vi "Find Array High-Low Levels.vi"(8 "Error In":errorcluster, 9 "Method (Mode)":T1, 10 "# Bins (auto)":i32, 11 "Array":dbl[](array[numeric])) -> (0 "Error Out":errorcluster, 1 "Low Level":dbl format="%0.2f", 3 "High Level":dbl format="%0.2f")   [LabVIEW 2021, in "Arrays.lvlib"]
doc: "Split the array into its lower and higher 50 percentiles and computes the mode (or mean) of each part."
uses:
  Arrays.lvlib
  Fits/Square Pulse/Square Pulse Levels Type.ctl
  Histograms/Histogram Bin Position.ctl
  Histograms/Linear Histogram Options.ctl
  Histograms/Histogram Bin Option.ctl
  e09bfede-782a-433a-9cf0-25cc41a0cc0b.vi
  3c089a08-6f38-494f-b69c-1966d4ea5c7a.vi
  e09bfede-782a-433a-9cf0-25cc41a0cc0b.vi/e021cd17-e000-4244-b7f4-ec50548bdfcb.vi
  e09bfede-782a-433a-9cf0-25cc41a0cc0b.vi/b1828c6e-eb0a-43e9-a724-8b596c52e435.vi
  e09bfede-782a-433a-9cf0-25cc41a0cc0b.vi/7a6138ed-c001-4311-b538-9ba42ae7c7b1.vi
  e09bfede-782a-433a-9cf0-25cc41a0cc0b.vi/52c6b4fa-501b-4af0-803b-8bab516ca5d3.vi
  e09bfede-782a-433a-9cf0-25cc41a0cc0b.vi/d7237e10-35ab-4bcb-a0c6-4883c3f4c990.vi
  e09bfede-782a-433a-9cf0-25cc41a0cc0b.vi/5fb5dd96-3b97-4592-ba56-58181c8e7105.vi
  e09bfede-782a-433a-9cf0-25cc41a0cc0b.vi/8e13a849-a393-4484-9968-4af7b25c38d7.vi
  3c089a08-6f38-494f-b69c-1966d4ea5c7a.vi/e021cd17-e000-4244-b7f4-ec50548bdfcb.vi
  3c089a08-6f38-494f-b69c-1966d4ea5c7a.vi/b1828c6e-eb0a-43e9-a724-8b596c52e435.vi
  3c089a08-6f38-494f-b69c-1966d4ea5c7a.vi/7a6138ed-c001-4311-b538-9ba42ae7c7b1.vi
  3c089a08-6f38-494f-b69c-1966d4ea5c7a.vi/52c6b4fa-501b-4af0-803b-8bab516ca5d3.vi
  3c089a08-6f38-494f-b69c-1966d4ea5c7a.vi/d7237e10-35ab-4bcb-a0c6-4883c3f4c990.vi
  3c089a08-6f38-494f-b69c-1966d4ea5c7a.vi/5fb5dd96-3b97-4592-ba56-58181c8e7105.vi
  3c089a08-6f38-494f-b69c-1966d4ea5c7a.vi/8e13a849-a393-4484-9968-4af7b25c38d7.vi
  Time/High Resolution Timing.vi
  <userlib>/_OpenG.lib/array/array.llb/Filter 1D Array__ogtk.vi
  <userlib>/_OpenG.lib/array/array.llb/Filter 1D Array (DBL)__ogtk.vi
  <userlib>/_OpenG.lib/array/array.llb/Delete Elements from Array__ogtk.vi
  <userlib>/_OpenG.lib/array/array.llb/Delete Elements from 1D Array (DBL)__ogtk.vi
  <vilib>/Utility/error.llb/Error Cluster From Error Code.vi
  Histograms/Histogram Window.lvlib
  Math/Math.lvlib
  Fits/Fits.lvlib
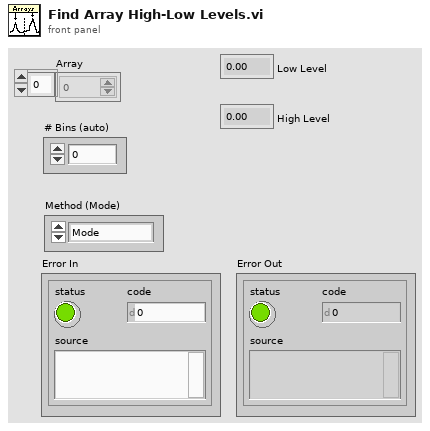
[diagram p1: front panel]
types:
  T1 = typedef "Fits.lvlib/Square Pulse Levels Type.ctl" = enum16{"Mode", "Mean"}
  T2 = typedef "Histogram Window.lvlib/Histogram Bin Option.ctl" = enum32{"Bin Number", "Bin Size"}
  T3 = typedef "Histogram Window.lvlib/Linear Histogram Options.ctl" = cluster{"Bin Size":dbl, "Bin Number":i32, "Bin Option":T2, "Min Value":dbl, "Max Value":dbl, "Filter NaN & Infinite Values":bool, "Frequency Plot":bool, "Align Bins":bool, "Bin Location":T4, "Project Outside Values":bool, "Max Histogram Size":i32}
  T4 = typedef "Histogram Window.lvlib/Histogram Bin Position.ctl" = enum16{"Left", "Center", "Right"}
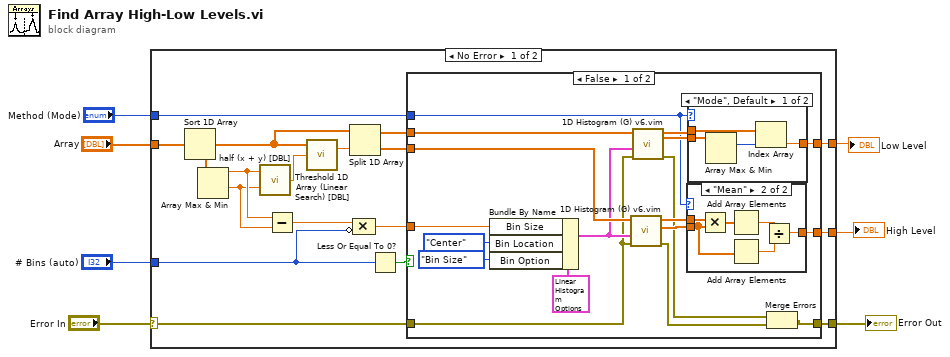
[diagram p0: block diagram]
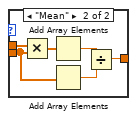
[diagram p2: hidden frame]
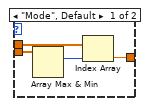
[diagram p3: hidden frame]
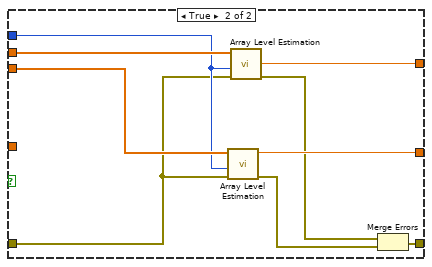
[diagram p4: hidden frame]
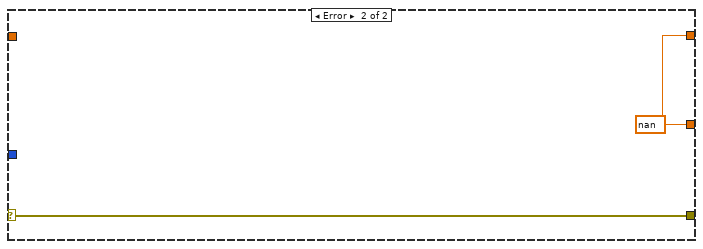
[diagram p5: hidden frame]
diagram:
  n1 = case shown="No Error" "Error In" {
    selector: "Error In" -> [w9 w73]
    tunnel: "Array" -> [w24 _]
    tunnel: [w22 w72] -> w6
    tunnel: [w21 w72] -> w5
    tunnel: "# Bins (auto)" -> [w18 _]
    tunnel: "Method (Mode)" -> [w13 _]
    tunnel: [w8 w73] -> w1
    frame No Error {
      n2 = Sort 1D Array(array=w24) -> (sorted array=w20:dbl[])
      n3 = Array Max & Min(array=w20) -> (max value=w12:dbl, min value=w11:dbl)  [unwired: 2 out]
      n4 = call "half (x + y) [DBL].vi"("y"=w11, "x"=w12) -> ("(x+y)/2"=w10:dbl)  [unwired: 4 in]
      n5 = Subtract(x=w12, y=w11) -> (x-y=w19:dbl)
      n6 = call "Threshold 1D Array (Linear Search) [DBL].vi"("Array"=w20, "Y"=w10) -> ("fractional index"=w23:dbl)  [unwired: 7 in]
      n7 = Split 1D Array(array=w20, index=w23) -> (first subarray=w14:dbl[], second subarray=w17:dbl[])
      n8 = Compound Arithmetic op=MULTIPLY(w19, invert w18) -> (w16:dbl)
      n9 = Less Or Equal To 0?(x=w18) -> (x <= 0?=w15:bool)
      n10 = case shown="False" w15 {
        tunnel: [w42 w70] -> w22
        tunnel: [w41 w71] -> w21
        tunnel: w14 -> [w36 w69]
        tunnel: w13 -> [w35 w67]
        tunnel: w17 -> [w34 w68]
        tunnel: w16 -> [w32 _]
        tunnel: w9 -> [w29 w66]
        tunnel: [w26 w63] -> w8
        frame False {
          n11 = Bundle By Name(cluster=T3 {"Bin Size"=nan, "Bin Number"=0, "Bin Option"=enum."Bin Number", "Min Value"=-inf, "Max Value"=inf, "Filter NaN & Infinite Values"=FALSE, "Frequency Plot"=FALSE, "Align Bins"=FALSE, "Bin Location"=enum."Left", "Project Outside Values"=FALSE, "Max Histogram Size"=100000} ("Histogram Options"), "Bin Size"=w32, "Bin Location"=Histogram_Bin_Position."Center" ("Bin Location (Left)"), "Bin Option"=Histogram_Bin_Option."Bin Size" ("Bin Size")) -> (w30:T3)
          n12 = call "1D Histogram (G) v6.vim"("Error In"=w29, "Histogram Options"=w30, "Array"=w34) -> ("Error Out"=w27:errorcluster, "Histogram"=w37:dbl[], "Axis"=w38:dbl[])  [unwired: 2 in, 4 out]
          n13 = call "1D Histogram (G) v6.vim"("Error In"=w29, "Histogram Options"=w30, "Array"=w36) -> ("Error Out"=w28:errorcluster, "Histogram"=w39:dbl[], "Axis"=w40:dbl[])  [unwired: 2 in, 4 out]
          n14 = case shown="\"Mean\"" w35 {
            tunnel: w37 -> [w56 w60]
            tunnel: w38 -> [w55 w62]
            tunnel: [w53 w57] -> w42
            frame "Mode", Default {
              n15 = Array Max & Min(array=w56) -> (max index (indices)=w54:i32)  [unwired: 3 out]
              n16 = Index Array(array=w55, index=w54) -> (element=w53:dbl)
            }
            frame "Mean" {
              n17 = Multiply(x=w62, y=w60) -> (x*y=w61:dbl[])
              n18 = Add Array Elements(numeric array=w61) -> (sum=w59:dbl)
              n19 = Add Array Elements(numeric array=w60) -> (sum=w58:dbl)
              n20 = Divide(x=w59, y=w58) -> (x/y=w57:dbl)
            }
          }
          n21 = case shown="\"Mode\", Default" w35 {
            tunnel: w39 -> [w46 w50]
            tunnel: w40 -> [w45 w52]
            tunnel: [w43 w47] -> w41
            frame "Mode", Default {
              n22 = Array Max & Min(array=w46) -> (max index (indices)=w44:i32)  [unwired: 3 out]
              n23 = Index Array(array=w45, index=w44) -> (element=w43:dbl)
            }
            frame "Mean" {
              n24 = Multiply(x=w52, y=w50) -> (x*y=w51:dbl[])
              n25 = Add Array Elements(numeric array=w51) -> (sum=w49:dbl)
              n26 = Add Array Elements(numeric array=w50) -> (sum=w48:dbl)
              n27 = Divide(x=w49, y=w48) -> (x/y=w47:dbl)
            }
          }
          n28 = Merge Errors(w28, w27) -> (w26:errorcluster)
        }
        frame True {
          n29 = call "Array Level Estimation.vi"("Error In"=w66, "Method (Mode)"=w67, "Array"=w68) -> ("Error Out"=w65:errorcluster, "Level"=w70:dbl)  [unwired: 7 in]
          n30 = call "Array Level Estimation.vi"("Error In"=w66, "Method (Mode)"=w67, "Array"=w69) -> ("Error Out"=w64:errorcluster, "Level"=w71:dbl)  [unwired: 7 in]
          n31 = Merge Errors(w64, w65) -> (w63:errorcluster)
        }
      }
    }
    frame Error {
      w72 = nan ("Level")
    }
  }
  "Low Level" <- w5
  "High Level" <- w6
  "Error Out" <- w1
